vi "2-Sine Wave Chart (while loop with continue if true).vi"() -> ()   [LabVIEW 2014]
panel:
  in  "stop":bool
  out "Waveform Chart":dbl(graph)
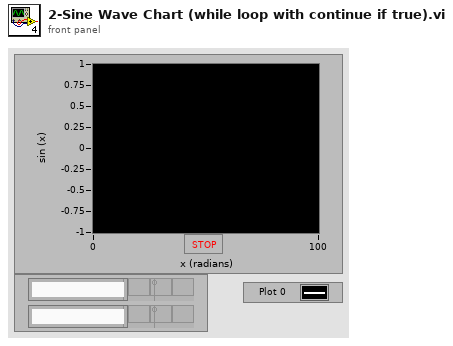
[diagram p1: front panel]
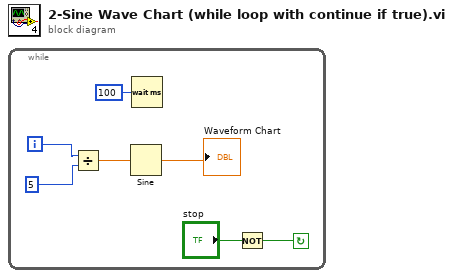
[diagram p0: block diagram]
diagram:
  n1 = while {
    i -> [w5]
    stop <- w1 continue-if-true
    n2 = Divide(x=w5, y=5) -> (x/y=w7:dbl)
    n3 = Sine(x=w7) -> (sin(x)=→"Waveform Chart":dbl)
    n4 = Wait (ms)(milliseconds to wait=u32 100) -> ()  [unwired: 1 out]
    n5 = Not(x="stop") -> (.not. x?=w1:bool)
  }
